vi "perform_piecewise_function.vi"(6 "function array":dbl[][](array[numeric]), 10 "x":T1) -> (2 "y":T1)   [LabVIEW 2020]
uses:
  <vilib>/Analysis/Matrix/Datatypes/RealMatrix.ctl
  <vilib>/Analysis/Matrix/Numeric/Conversions/Array To Matrix - RA.vi
  <vilib>/Analysis/Matrix/NI_Matrix.lvlib
panel:
  out "Array":dbl[](array[numeric])
  out "indicator":dbl
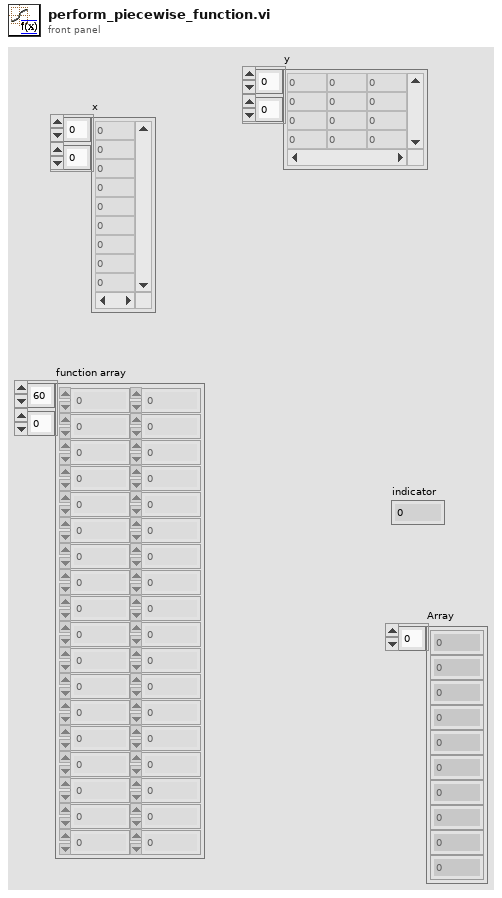
[diagram p1: front panel]
types:
  T1 = typedef "NI_Matrix.lvlib/RealMatrix.ctl" = dbl[][]
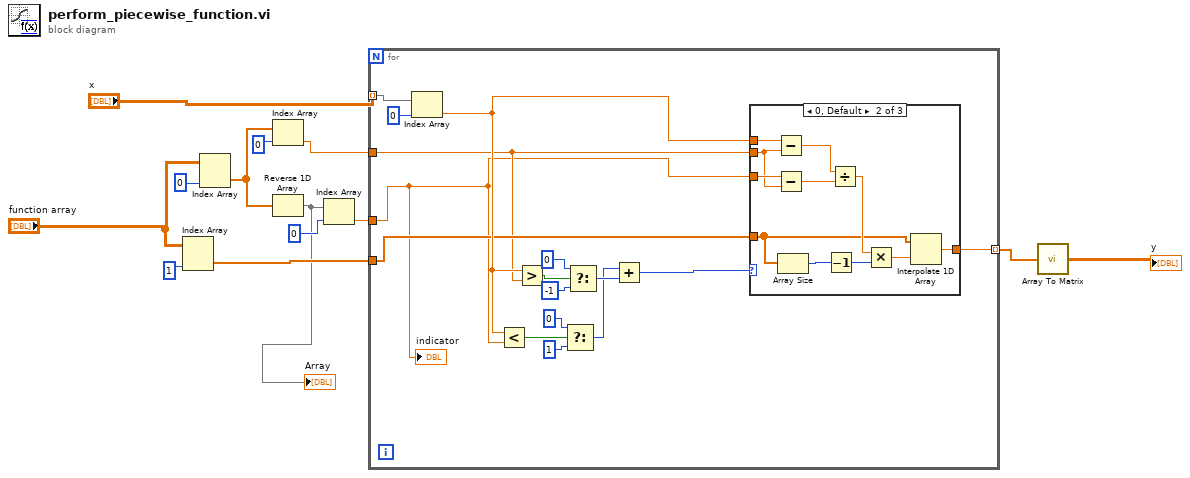
[diagram p0: block diagram]
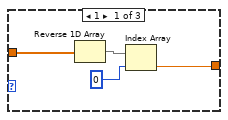
[diagram p2: hidden frame]
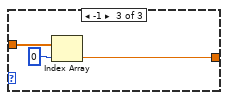
[diagram p3: hidden frame]
diagram:
  n1 = Index Array(array="function array", index (col)=1) -> (element=w8:dbl[])  [unwired: 1 in]
  n2 = Index Array(array="function array", index (col)=0) -> (element=w3:dbl[])  [unwired: 1 in]
  n3 = Index Array(array=w3, index=0) -> (element=w4:dbl)
  n4 = Reverse 1D Array(array=w3) -> (reversed array=w1:dbl[])
  "Array" <- w1
  n5 = Index Array(array=w1, index=0) -> (element=w5:dbl)
  n6 = for {
    tunnel: w4 -> [w16]
    tunnel: [w29] -> w12 mode=indexing
    tunnel: "x" -> [w20] mode=indexing
    tunnel: w8 -> [w17]
    tunnel: w5 -> [w14]
    n7 = Index Array(array=w20, index=0) -> (element=w18:dbl)
    n8 = Less?(x=w18, y=w14) -> (x < y?=w24:bool)
    n9 = Greater?(x=w18, y=w16) -> (0:w21:bool)
    n10 = Select(t=0, s=w24, f=1) -> (s? t:f=w27:i32)
    n11 = Select(t=0, s=w21, f=-1) -> (s? t:f=w28:i32)
    n12 = Add(x=w27, y=w28) -> (x+y=w15:i32)
    n13 = case shown="0, Default" w15 {
      tunnel: w17 -> [w31 w37 w47]
      tunnel: [w30 w36 w45] -> w29
      tunnel: w18 -> [_ w44 _]
      tunnel: w16 -> [_ w42 _]
      tunnel: w14 -> [_ w43 _]
      frame 1 {
        n14 = Reverse 1D Array(array=w31) -> (reversed array=w33:dbl[])
        n15 = Index Array(array=w33, index=0) -> (element=w30:dbl)
      }
      frame 0, Default {
        n16 = Subtract(x=w44, y=w42) -> (x-y=w41:dbl)
        n17 = Subtract(x=w43, y=w42) -> (x-y=w40:dbl)
        n18 = Array Size(array=w37) -> (size(s)=w35:i32)
        n19 = Decrement(x=w35) -> (x-1=w34:i32)
        n20 = Divide(x=w41, y=w40) -> (x/y=w39:dbl)
        n21 = Multiply(x=w39, y=w34) -> (x*y=w38:dbl)
        n22 = Interpolate 1D Array(1:w38, 2:w37) -> (0:w36:dbl)
      }
      frame -1 {
        n23 = Index Array(array=w47, index=0) -> (element=w45:dbl)
      }
    }
    "indicator" <- w14
  }
  n24 = call-poly <vilib>:"Array To Matrix.vi"("Real 1D Array"=w12) -> ("Real Matrix (Column Vector)"=→"y":T1)
